vi "ROI entry-Offset limits.vi"(9 "Offsets cluster in in":cluster{"X offset":dbl, "Y offset":dbl}, 10 "Function":T1=enum."Offset all ROI", 11 "ROI setup in":T2[](array[typedef]) {"ROI group ID" format="%#_6f"; "Laser Power (%)" format="%#_6f"; "Zoom" format="%#_6f"; "Frame Size" format="%#_6f"; "Number of lines" format="%#_6f"; "Composite ID" format="%#_6f"; "Angle (deg)" format="%#_6f"; "ROI Time (ns)" format="%#_6f"; "ROI ID" format="%#_6f"; "Pixels in ROI" format="%#_6f"; "ROI index" format="%#_6f"; "Z stop" format="%#_6f"; "Y stop" format="%#_6f"; "X stop" format="%#_6f"; "Z start" format="%#_6f"; "X start" format="%#_6f"; "Y start" format="%#_6f"}) -> (3 "Offsets cluster out":T3)   [LabVIEW 2013]
uses:
  Typedefs/Offset adjustments cluster.ctl
  Visualisation/Functional Imaging Viewer/Typedefs/ROI parameters data type.ctl
  Typedefs/ROI management FG states.ctl
  Program Files (x86)/National Instruments/LabVIEW 2013/user.lib/_OpenG.lib/array/array.llb/Conditional Auto-Indexing Tunnel (DBL)__ogtk.vi
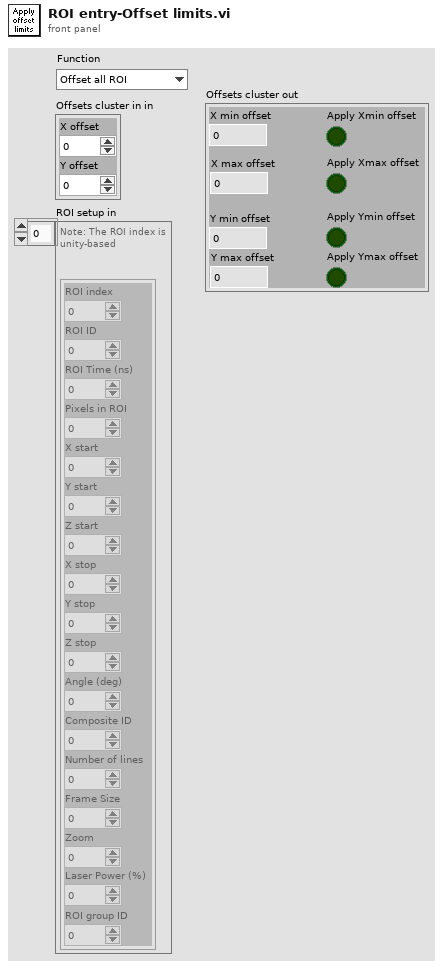
[diagram p1: front panel]
types:
  T1 = typedef "ROI management FG states.ctl" = enum16{"Read", "Write", "Clear Last", "Clear All", "Update ROIs time", "Reload last ROI set", "Offset all ROI", "Offset visible ROI"}
  T2 = typedef "ROI parameters data type.ctl" = cluster{"ROI index":dbl, "ROI ID":dbl, "ROI Time (ns)":dbl, "Pixels in ROI":dbl, "X start":dbl, "Y start":dbl, "Z start":dbl, "X stop":dbl, "Y stop":dbl, "Z stop":dbl, "Angle (deg)":dbl, "Composite ID":dbl, "Number of lines":dbl, "Frame Size":dbl, "Zoom":dbl, "Laser Power (%)":dbl, "ROI group ID":dbl}
  T3 = typedef "Offset adjustments cluster.ctl" = cluster{"X min offset":dbl, "Apply Xmin offset":bool, "X max offset":dbl, "Apply Xmax offset":bool, "Y min offset":dbl, "Apply Ymin offset":bool, "Y max offset":dbl, "Apply Ymax offset":bool}
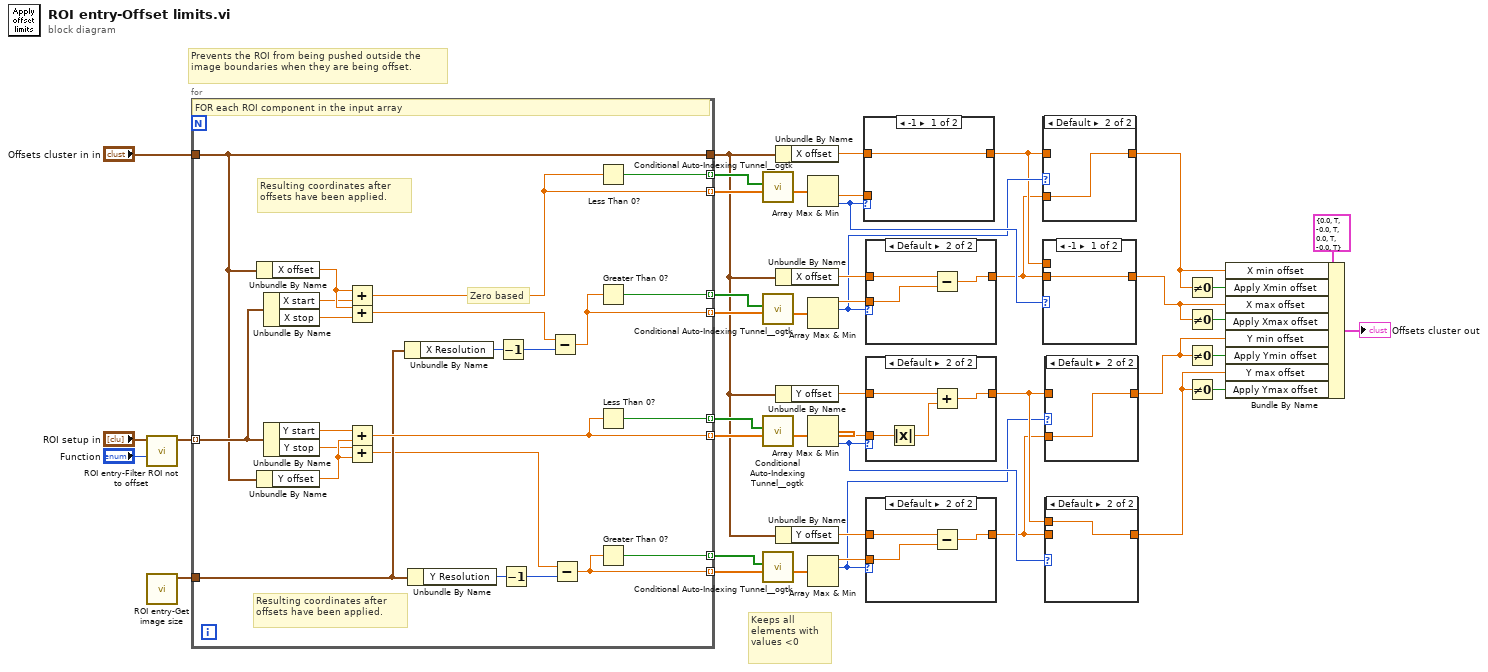
[diagram p0: block diagram]
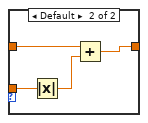
[diagram p9: hidden frame]
diagram:
  # "Keeps all elements with values <0"
  # "Prevents the ROI from being pushed outside the image boundaries when they are being offset."
  n1 = call "ROI entry-Filter ROI not to offset.vi"("Function"="Function", "ROI setup in"="ROI setup in") -> ("Filtered ROI"=w2:T2[])  [unwired: 9 in]
  n2 = call "ROI entry-Get image size.vi"() -> ("Image size"=w43:cluster{"X Resolution":i32, "Y Resolution":i32})  [unwired: 10 in, 1 out]
  n3 = for {
    tunnel: "Offsets cluster in in" -> [w49]
    tunnel: w2 -> [w56] mode=indexing
    tunnel: [w49] -> w21
    tunnel: [w55] -> w37 mode=indexing
    tunnel: [w50] -> w38 mode=indexing
    tunnel: [w60] -> w40 mode=indexing
    tunnel: [w62] -> w42 mode=indexing
    tunnel: w43 -> [w52]
    tunnel: [w61] -> w41 mode=indexing
    tunnel: [w59] -> w39 mode=indexing
    tunnel: [w54] -> w36 mode=indexing
    tunnel: [w51] -> w35 mode=indexing
    # "Resulting coordinates after offsets have been applied."
    # "Resulting coordinates after offsets have been applied."
    # "Zero based"
    # "FOR each ROI component in the input array"
    n4 = Unbundle By Name(w49) -> ("X offset"=w67:dbl)
    n5 = Unbundle By Name(w49) -> ("Y offset"=w66:dbl)
    n6 = Unbundle By Name(w56) -> ("X start"=w58:dbl, "X stop"=w57:dbl)
    n7 = Unbundle By Name(w56) -> ("Y start"=w65:dbl, "Y stop"=w64:dbl)
    n8 = Add(x=w67, y=w58) -> (x+y=w55:dbl)
    n9 = Add(x=w67, y=w57) -> (x+y=w45:dbl)
    n10 = Add(x=w65, y=w66) -> (x+y=w60:dbl)
    n11 = Add(x=w64, y=w66) -> (x+y=w48:dbl)
    n12 = Unbundle By Name(w52) -> ("X Resolution"=w53:i32)
    n13 = Unbundle By Name(w52) -> ("Y Resolution"=w63:i32)
    n14 = Decrement(x=w53) -> (x-1=w46:i32)
    n15 = Decrement(x=w63) -> (x-1=w47:i32)
    n16 = Subtract(x=w45, y=w46) -> (x-y=w50:dbl)
    n17 = Subtract(x=w48, y=w47) -> (x-y=w62:dbl)
    n18 = Less Than 0?(x=w55) -> (x < 0?=w54:bool)
    n19 = Greater Than 0?(x=w50) -> (x > 0?=w51:bool)
    n20 = Less Than 0?(x=w60) -> (x < 0?=w59:bool)
    n21 = Greater Than 0?(x=w62) -> (x > 0?=w61:bool)
  }
  n22 = call-poly "Conditional Auto-Indexing Tunnel__ogtk.vi"("Array in"=w37, "Elements to keep"=w36) -> ("Filtered Array out"=w33:dbl[])  [unwired: 5 in]
  n23 = call-poly "Conditional Auto-Indexing Tunnel__ogtk.vi"("Array in"=w38, "Elements to keep"=w35) -> ("Filtered Array out"=w30:dbl[])  [unwired: 5 in]
  n24 = call-poly "Conditional Auto-Indexing Tunnel__ogtk.vi"("Array in"=w40, "Elements to keep"=w39) -> ("Filtered Array out"=w31:dbl[])  [unwired: 5 in]
  n25 = call-poly "Conditional Auto-Indexing Tunnel__ogtk.vi"("Array in"=w42, "Elements to keep"=w41) -> ("Filtered Array out"=w29:dbl[])  [unwired: 5 in]
  n26 = Unbundle By Name(w21) -> ("X offset"=w24:dbl)
  n27 = Unbundle By Name(w21) -> ("X offset"=w20:dbl)
  n28 = Unbundle By Name(w21) -> ("Y offset"=w23:dbl)
  n29 = Unbundle By Name(w21) -> ("Y offset"=w18:dbl)
  n30 = Array Max & Min(array=w33) -> (min value=w32:dbl, min index (indices)=w16:i32)  [unwired: 2 out]
  n31 = Array Max & Min(array=w30) -> (max value=w19:dbl, max index (indices)=w14:i32)  [unwired: 2 out]
  n32 = Array Max & Min(array=w31) -> (min value=w22:dbl, min index (indices)=w9:i32)  [unwired: 2 out]
  n33 = Array Max & Min(array=w29) -> (max value=w17:dbl, max index (indices)=w7:i32)  [unwired: 2 out]
  n34 = case shown="-1" w16 {
    tunnel: w32 -> [_ w72]
    tunnel: [w68 w69] -> w13
    tunnel: w24 -> [w68 w70]
    frame -1 {
    }
    frame Default {
      n35 = Absolute Value(x=w72) -> (abs(x)=w71:dbl)
      n36 = Add(x=w70, y=w71) -> (x+y=w69:dbl)
    }
  }
  n37 = case shown="Default" w14 {
    tunnel: [w73 w75] -> w12
    tunnel: w20 -> [w73 w76]
    tunnel: w19 -> [_ w74]
    frame -1 {
    }
    frame Default {
      n38 = Subtract(x=w76, y=w74) -> (x-y=w75:dbl)
    }
  }
  n39 = case shown="Default" w9 {
    tunnel: w22 -> [_ w81]
    tunnel: [w77 w78] -> w8
    tunnel: w23 -> [w77 w79]
    frame -1 {
    }
    frame Default {
      n40 = Absolute Value(x=w81) -> (abs(x)=w80:dbl)
      n41 = Add(x=w79, y=w80) -> (x+y=w78:dbl)
    }
  }
  n42 = case shown="Default" w7 {
    tunnel: [w82 w84] -> w6
    tunnel: w18 -> [w82 w85]
    tunnel: w17 -> [_ w83]
    frame -1 {
    }
    frame Default {
      n43 = Subtract(x=w85, y=w83) -> (x-y=w84:dbl)
    }
  }
  n44 = case shown="Default" w14 {
    tunnel: w13 -> [w86 _]
    tunnel: [w86 w87] -> w5
    tunnel: w12 -> [_ w87]
    frame -1 {
    }
    frame Default {
    }
  }
  n45 = case shown="-1" w16 {
    tunnel: w12 -> [w88 _]
    tunnel: [w88 w89] -> w15
    tunnel: w13 -> [_ w89]
    frame -1 {
    }
    frame Default {
    }
  }
  n46 = case shown="Default" w7 {
    tunnel: w8 -> [w90 _]
    tunnel: [w90 w91] -> w11
    tunnel: w6 -> [_ w91]
    frame -1 {
    }
    frame Default {
    }
  }
  n47 = case shown="Default" w9 {
    tunnel: w6 -> [w92 _]
    tunnel: [w92 w93] -> w10
    tunnel: w8 -> [_ w93]
    frame -1 {
    }
    frame Default {
    }
  }
  n48 = Not Equal To 0?(x=w5) -> (x != 0?=w28:bool)
  n49 = Not Equal To 0?(x=w15) -> (x != 0?=w27:bool)
  n50 = Not Equal To 0?(x=w11) -> (x != 0?=w25:bool)
  n51 = Not Equal To 0?(x=w10) -> (x != 0?=w26:bool)
  n52 = Bundle By Name(cluster=T3 {"X min offset"=0.0, "Apply Xmin offset"=TRUE, "X max offset"=-0.0, "Apply Xmax offset"=TRUE, "Y min offset"=0.0, "Apply Ymin offset"=TRUE, "Y max offset"=-0.0, "Apply Ymax offset"=TRUE} ("Offsets cluster out"), "X min offset"=w5, "Apply Xmin offset"=w28, "X max offset"=w15, "Apply Xmax offset"=w27, "Y min offset"=w11, "Apply Ymin offset"=w25, "Y max offset"=w10, "Apply Ymax offset"=w26) -> (→"Offsets cluster out":T3)
